vi "get_enabled_state.vi"(8 "error in (no error)":errorcluster, 11 "GenericStimulator in":refnum<class "GenericStimulator.lvclass">) -> (0 "error out":errorcluster, 2 "stimulator enabled?":bool, 3 "GenericStimulator out":refnum<class "GenericStimulator.lvclass">)   [LabVIEW 2010, in "GenericStimulator.lvclass"]
doc: "returns the boolean flag indicating whether or not stimulator functionality is enabled (value set on on the stimulator tab of the main VI front panel)"
uses:
  GenericStimulator.lvclass
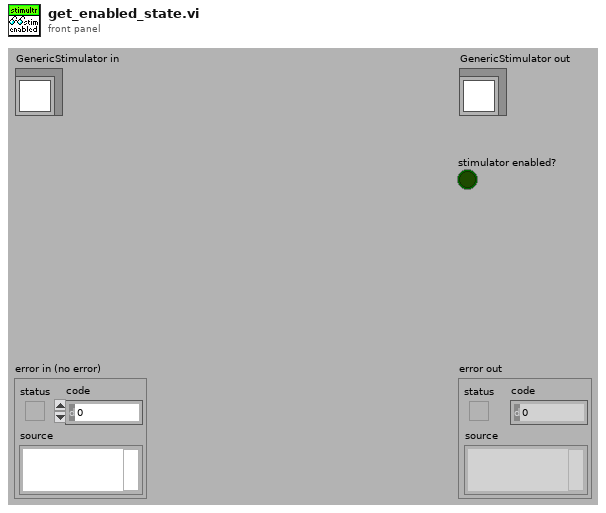
[diagram p1: front panel]
types:
  T1 = typedef "controls_refs.ctl" = cluster{"buttons":cluster{"start_focus":refnum<vi>, "start_single_sweep":refnum<vi>, "start_experiment":refnum<vi>, "save":refnum<vi>, "exit":refnum<vi>}, "tabs":cluster{"main":refnum<vi>, "settings":refnum<vi>}, "subpanels":cluster{"imagingMode":refnum<vi>, "scanHead":refnum<vi>, "display":refnum<vi>, "experimentController":refnum<vi>, "instrument":refnum<vi>, "stage":refnum<vi>, "stimulator":refnum<vi>, "dataCollection":refnum<vi>, "analyser":refnum<vi>, "daq":refnum<vi>, "imageAssembler":refnum<vi>}, "drop-downs":cluster{"imagingMode":refnum<vi>, "experimentalController":refnum<vi>, "objective":refnum<vi>}, "status lights":cluster{"experimentController":refnum<vi>, "imagingMode":refnum<vi>, "scanHead":refnum<vi>, "daq":refnum<vi>, "imageAssembler":refnum<vi>, "dataCollection":refnum<vi>, "display":refnum<vi>, "analyser":refnum<vi>, "stage":refnum<vi>, "stimulator":refnum<vi>, "instrument":refnum<vi>}, "message":refnum<vi>, "stimulator enabled?":refnum<vi>, "saving":cluster{"data folder path":refnum<vi>, "file base name":refnum<vi>, "notebook":refnum<vi>}, "progress bar":refnum<vi>, "update icon":refnum<vi>, "title":refnum<vi>, "main vi":refnum<vi>, "user":refnum<vi>}
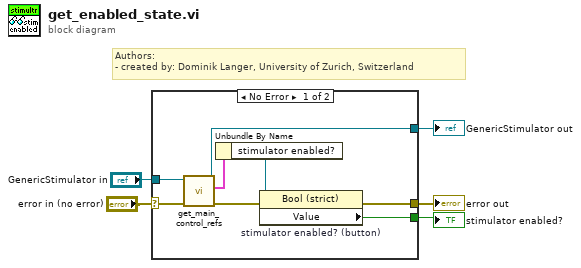
[diagram p0: block diagram]
diagram:
  # "Authors: \n- created by: Dominik Langer, University of Zurich, Switzerland"
  n1 = case shown="No Error" "error in (no error)" {
    selector: "error in (no error)" -> [w13 w15]
    tunnel: [w7 w15] -> w4
    tunnel: [w11 w14] -> w2
    tunnel: "GenericStimulator in" -> [w12 w14]
    tunnel: [w6 _] -> w1
    frame No Error {
      n2 = call-dynamic "get_main_control_refs.vi"("error in (no error)"=w13, "GenericPlugin.lvclass in"=w12) -> ("error out"=w8:errorcluster, "control references"=w10:T1, "GenericPlugin.lvclass out"=w11:refnum<class "GenericStimulator.lvclass">)  [unwired: 7 in]
      n3 = Unbundle By Name(w10) -> ("stimulator enabled?"=w9:refnum<vi>)
      n4 = property on="stimulator enabled? (button)" class="Bool (strict)"(reference=w9, error in=w8) -> (error out=w7:errorcluster, "Value"=w6:bool)  [unwired: 1 out]
    }
    frame Error {
    }
  }
  "error out" <- w4
  "GenericStimulator out" <- w2
  "stimulator enabled?" <- w1
